vi "Create Metadata Response.vi"(8 "error in":errorcluster, 9 "gRPC ID":T9, 10 "measurement plugin service in":refnum<class "Measurement Plugin Service.lvclass">) -> (0 "error out":errorcluster, 2 "get metadata response":T1, 3 "gRPC ID out":T9)   [LabVIEW 2021, in "NI Measurement Plug-In SDK.lvlib" / "IMeasurement Service.lvclass"]
uses:
  IMeasurement Service.lvclass
  <vilib>/gRPC/LabVIEW gRPC Library/Shared/grpcId.ctl
  Helpers/TypeDefs/Get Metadata Response.ctl
  Helpers/TypeDefs/Measurement Details.ctl
  Helpers/TypeDefs/Measurement Signature.ctl
  Helpers/TypeDefs/Configuration Parameter.ctl
  Helpers/TypeDefs/Parameter Annotations Entry.ctl
  <vilib>/gRPC/LabVIEW gRPC Library/Shared/Any.ctl
  Helpers/TypeDefs/Output Parameter.ctl
  Helpers/TypeDefs/User Interface Details.ctl
  Measurement Plugin Service/Measurement Plugin Service.lvclass
  <vilib>/gRPC/LabVIEW gRPC Library/Server API/typeDefs/gRPC Status Code.ctl
  NI Measurement Plug-In SDK.lvlib
  <vilib>/gRPC/LabVIEW gRPC Library/grpc-lvsupport-release.lvlib
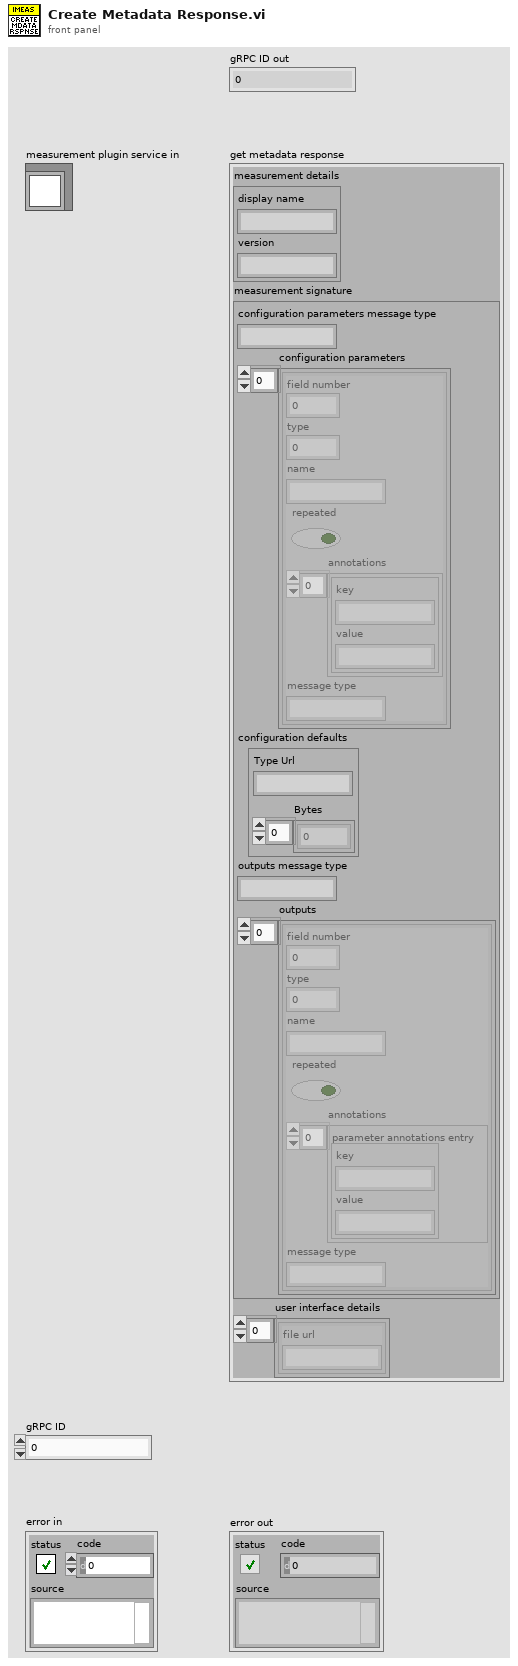
[diagram p1: front panel]
types:
  T1 = typedef "NI Measurement Plug-In SDK.lvlib/Get Metadata Response.ctl" = cluster{"measurement details":T2, "measurement signature":T3, "user interface details":T8[]}
  T2 = typedef "NI Measurement Plug-In SDK.lvlib/Measurement Details.ctl" = cluster{"display name":string, "version":string}
  T3 = typedef "NI Measurement Plug-In SDK.lvlib/Measurement Signature.ctl" = cluster{"configuration parameters message type":string, "configuration parameters":T4[], "configuration defaults":T6, "outputs message type":string, "outputs":T7[]}
  T4 = typedef "NI Measurement Plug-In SDK.lvlib/Configuration Parameter.ctl" = cluster{"field number":i32, "type":i32, "name":string, "repeated":bool, "annotations":T5[], "message type":string}
  T5 = typedef "NI Measurement Plug-In SDK.lvlib/Parameter Annotations Entry.ctl" = cluster{"key":string, "value":string}
  T6 = typedef "grpc-lvsupport-release.lvlib/Any.ctl" = cluster{"Type Url":string, "Bytes":u8[]}
  T7 = typedef "NI Measurement Plug-In SDK.lvlib/Output Parameter.ctl" = cluster{"field number":i32, "type":i32, "name":string, "repeated":bool, "annotations":T5[], "message type":string}
  T8 = typedef "NI Measurement Plug-In SDK.lvlib/User Interface Details.ctl" = cluster{"file url":string}
  T9 = typedef "grpc-lvsupport-release.lvlib/grpcId.ctl" = u64
  T10 = typedef "grpc-lvsupport-release.lvlib/gRPC Status Code.ctl" = enum16{"OK", "CANCELLED", "UNKNOWN", "INVALID_ARGUMENT", "DEADLINE_EXCEEDED", "NOT_FOUND", "ALREADY_EXISTS", "PERMISSION_DENIED", "RESOURCE_EXHAUSTED", "FAILED_PRECONDITION", "ABORTED", "OUT_OF_RANGE", "UNIMPLEMENTED", "INTERNAL", "UNAVAILABLE", "DATA_LOSS", "UNAUTHENTICATED"}
  T11 = typedef "NI Measurement Plug-In SDK.lvlib/Measurement Plugin Service.lvclass/Plugin Paths.ctl" = cluster{"get service descriptor VI path":path, "get type specializations VI path":path, "get UI details VI path":path, "measurement logic VI path":path, "measurement configuration ctl path":path, "measurement results ctl path":path}
  T12 = typedef "NI Measurement Plug-In SDK.lvlib/Service Descriptor.ctl" = cluster{"measurement details":T2, "description URL":string, "service class":string, "measurement annotations":T13[]}
  T13 = typedef "NI Measurement Plug-In SDK.lvlib/Measurement Annotation.ctl" = cluster{"key":string, "value":string}
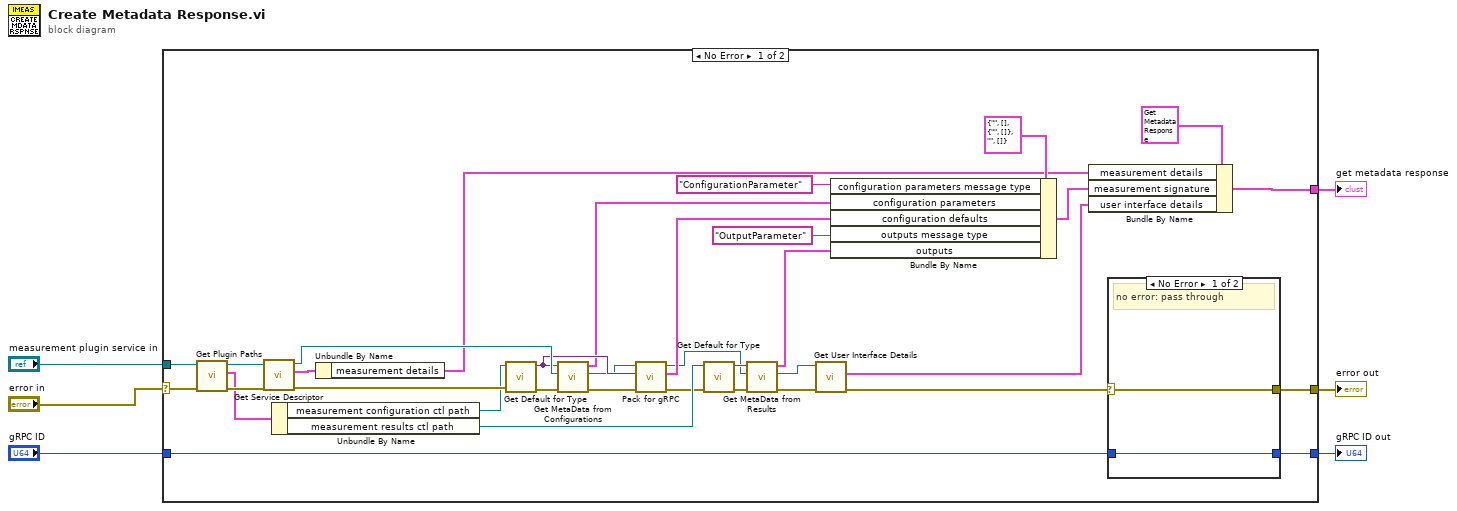
[diagram p0: block diagram]
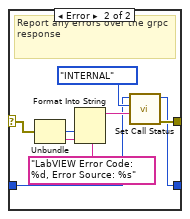
[diagram p2: hidden frame]
diagram:
  n1 = case shown="No Error" "error in" {
    selector: "error in" -> [w12 w54]
    tunnel: [w37 w53] -> w6
    tunnel: "gRPC ID" -> [w36 w53]
    tunnel: [w35 w54] -> w4
    tunnel: [w33 _] -> w3
    tunnel: "measurement plugin service in" -> [w29 _]
    frame No Error {
      n2 = call-dynamic "Get Plugin Paths.vi"("error in"=w12, "measurement plugin service in"=w29) -> ("error out"=w40:errorcluster, "plugin paths"=w30:T11, "measurement plugin service out"=w38:refnum<class "Measurement Plugin Service.lvclass">)  [unwired: 7 in]
      n3 = call "Get Service Descriptor.vi"("error in"=w40, "measurement plugin service in"=w38) -> ("error out"=w41:errorcluster, "service descriptor"=w8:T12, "measurement plugin service out"=w39:refnum<class "Measurement Plugin Service.lvclass">)  [unwired: 7 in]
      n4 = Unbundle By Name(w30) -> ("measurement configuration ctl path"=w31:path, "measurement results ctl path"=w32:path)
      n5 = Unbundle By Name(w8) -> ("measurement details"=w7:T2)
      n6 = call "Get Default for Type.vi"("error in"=w41, "path of type"=w31) -> ("error out"=w18:errorcluster, "default for type"=w25:variant)  [unwired: 8 in]
      n7 = call "Get MetaData from Configurations.vi"("error in"=w18, "measurement plugin service in"=w39, "configuration cluster"=w25) -> ("error out"=w24:errorcluster, "measurement plugin service out"=w10:refnum<class "Measurement Plugin Service.lvclass">, "configuration parameters"=w13:T4[])  [unwired: 6 in]
      n8 = call-dynamic "Pack for gRPC.vi"("error in"=w24, "data value"=w25, "measurement plugin service in"=w10) -> ("error out"=w27:errorcluster, "any"=w26:T6, "measurement plugin service out"=w11:refnum<class "Measurement Plugin Service.lvclass">)  [unwired: 6 in]
      n9 = call "Get Default for Type.vi"("error in"=w27, "path of type"=w32) -> ("error out"=w23:errorcluster, "default for type"=w22:variant)  [unwired: 8 in]
      n10 = call "Get MetaData from Results.vi"("error in"=w23, "measurement plugin service in"=w11, "results cluster"=w22) -> ("error out"=w17:errorcluster, "measurement plugin service out"=w9:refnum<class "Measurement Plugin Service.lvclass">, "outputs"=w14:T7[])  [unwired: 6 in]
      n11 = call-dynamic "Get User Interface Details.vi"("error in"=w17, "measurement plugin service in"=w9) -> ("error out"=w34:errorcluster, "user interface details"=w28:T8[])  [unwired: 7 in, 1 out]
      n12 = Bundle By Name(cluster=T3 {"configuration parameters message type"="", "configuration parameters"=[], "configuration defaults"={"Type Url"="", "Bytes"=[]}, "outputs message type"="", "outputs"=[]} ("ni_measurements_v1_MeasurementSignature"), "configuration parameters message type"="ConfigurationParameter" ("configuration_parameters_messagetype"), "configuration parameters"=w13, "configuration defaults"=w26, "outputs message type"="OutputParameter" ("configuration_parameters_messagetype"), "outputs"=w14) -> (w20:T3)
      n13 = Bundle By Name(cluster=T1 {"measurement details"={"display name"="", "version"=""}, "measurement signature"={"configuration parameters message type"="", "configuration parameters"=[], "configuration defaults"={"Type Url"="", "Bytes"=[]}, "outputs message type"="", "outputs"=[]}, "user interface details"=[]} ("package_templatemessage"), "measurement details"=w7, "measurement signature"=w20, "user interface details"=w28) -> (w33:T1)
      n14 = case shown="No Error" w34 {
        selector: w34 -> [w42 w46]
        tunnel: [w42 w47] -> w35
        tunnel: w36 -> [w43 w45]
        tunnel: [w43 w44] -> w37
        frame No Error {
          # "no error: pass through"
        }
        frame Error {
          # "Report any errors over the grpc response"
          n15 = Unbundle(w46) -> ("code"=w50:i32, "source"=w51:string)  [unwired: 1 out]
          n16 = Format Into String(format string="LabVIEW Error Code: %d, Error Source: %s", w50, w51) -> (resulting string=w52:string)  [unwired: 2 in, 1 out]
          n17 = call <vilib>:"Set Call Status.vi"("Details"=w52, "Status Code"=gRPC_Status_Code."INTERNAL", "gRPCid in"=w45) -> ("error out"=w47:errorcluster, "gRPCid out"=w44:T9)  [unwired: 7 in]
        }
      }
    }
    frame Error {
    }
  }
  "gRPC ID out" <- w6
  "error out" <- w4
  "get metadata response" <- w3
